vi "lightmeter.vi"() -> ()   [LabVIEW 2020]
uses:
  <vilib>/LabVIEW Interface for Arduino/Type Defs/Board Type.ctl
  <vilib>/LabVIEW Interface for Arduino/Type Defs/Pin Mode.ctl
  <vilib>/LabVIEW Interface for Arduino/LabVIEW Interface for Arduino.lvlib
panel:
  out "With Averaging":cluster{"Y":dbl[], "Y":dbl[]}[](graph)
  out "error out":errorcluster
  # "Photodiode bias of GND\nLF411: Vcc of +/- 9V\nFeedback resistance of 10k Ohm\n100 Ohm Limiting resistor to white LED\nDark room to reduce background light\nProgramatically increase Duty cycle\nAveraging of 10 reads per data point"
  # "PWM_dutyCycle_LED.vi"
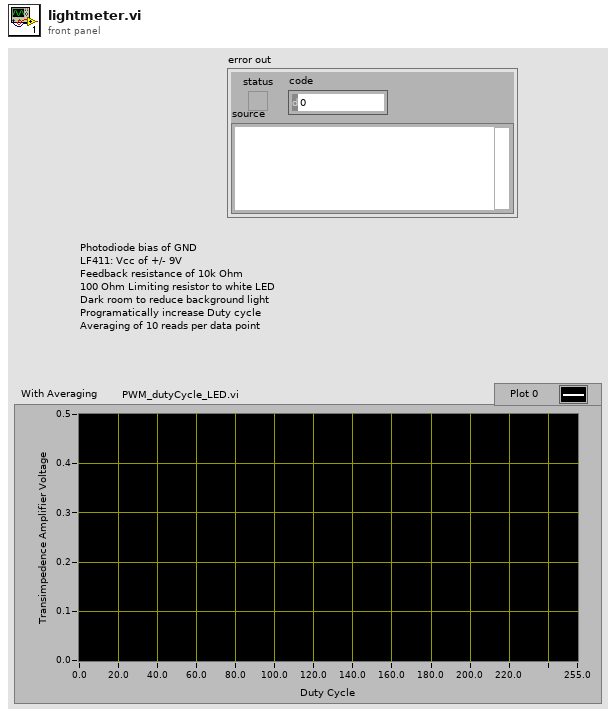
[diagram p1: front panel]
types:
  T1 = typedef "LabVIEW Interface for Arduino.lvlib/Pin Mode.ctl" = enum8{"Input", "Output"}
  T2 = typedef "LabVIEW Interface for Arduino.lvlib/Board Type.ctl" = enum16{"Uno", "Dimuelanove w/Atmega 328", "Mega 2560"}
  T3 = typedef "LabVIEW Interface for Arduino.lvlib/Arduino Resource.ctl" = cluster{"VISA resource":refnum<visa-resource-name>, "Board Type":T2, "Connection Type":enum8{"USB / Serial"}, "Bytes Per Packet (15)":u8}
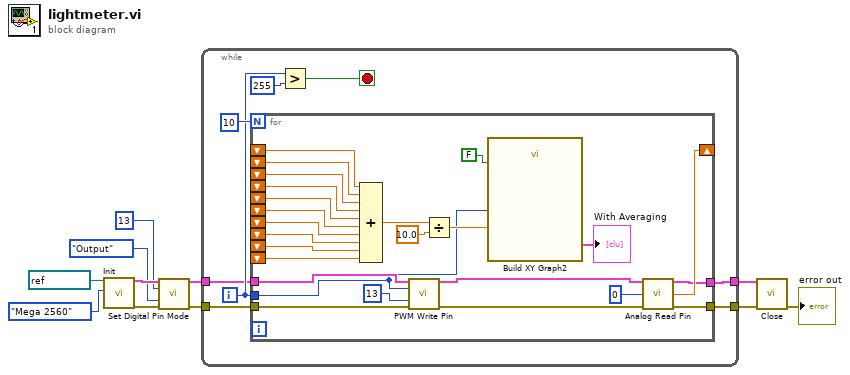
[diagram p0: block diagram]
diagram:
  n1 = call <vilib>:"Init.vi"("VISA resource"=refnum<visa-resource-name> "COM6", "Board Type (Uno)"=Board_Type."Mega 2560") -> ("Arduino Resource"=w10:T3, "error out"=w7:errorcluster)  [unwired: 16 in]
  n2 = call <vilib>:"Set Digital Pin Mode.vi"("Arduino Resource"=w10, "Digital I/O Pin"=u8 13, "Pin Mode (Input)"=Pin_Mode."Output", "error in"=w7) -> ("Arduino Resource"=w4:T3, "error out"=w3:errorcluster)  [unwired: 10 in]
  n3 = while {
    tunnel: w4 -> [w14]
    tunnel: w3 -> [w16]
    tunnel: [w13] -> w2
    tunnel: [w12] -> w1
    i -> [w15]
    stop <- w18 stop-if-true
    n4 = for {
      N: 10 -> [_]
      tunnel: [w44] -> w12
      tunnel: [w30] -> w13
      tunnel: w14 -> [w24]
      tunnel: w16 -> [w23]
      shift-right: [w43] -> _
      shift-left: _ -> [w42]
      shift-left: _ -> [w41]
      shift-left: _ -> [w40]
      shift-left: _ -> [w39]
      shift-left: _ -> [w38]
      shift-left: _ -> [w37]
      shift-left: _ -> [w36]
      shift-left: _ -> [w35]
      shift-left: _ -> [w34]
      shift-left: _ -> [w33]
      tunnel: w15 -> [w20]
      n5 = Compound Arithmetic op=ADD(w42, w41, w40, w39, w38, w37, w36, w35, w34, w33) -> (w31:dbl)
      n6 = call <vilib>:"PWM Write Pin.vi"("Arduino Resource"=w24, "Duty Cycle (0 - 255)"=w20, "PWM Pin (3)"=u8 13, "error in"=w23) -> ("Arduino Resource"=w21:T3, "error out"=w22:errorcluster)  [unwired: 10 in]
      n7 = Divide(x=w31, y=10.0) -> (x/y=w26:dbl)
      n8 = call "Build XY Graph2"("Reset"=FALSE, "Y Input"=w26, "X Input"=w20) -> ("XY Graph"=→"With Averaging":cluster{"X":dbl[], "Y":dbl[]}[])  [unwired: 7 in, 1 out]
      n9 = call <vilib>:"Analog Read Pin.vi"("Arduino Resource"=w21, "Analog Input Pin (0)"=u8 0 ("Digital I/O Pin (0)"), "error in"=w22) -> ("Arduino Resource"=w30:T3, "Voltage"=w43:dbl, "error out"=w44:errorcluster)  [unwired: 10 in]
    }
    n10 = Greater?(x=w15, y=255) -> (0:w18:bool)
  }
  n11 = call <vilib>:"Close.vi"("Arduino Resource"=w2, "error in"=w1) -> ("error out"=→"error out":errorcluster)  [unwired: 13 in]
